vi "Heat_global_variables.vi"() -> ()   [LabVIEW 2019]
uses:
  Monitors/Utility/Monitor Communication/K6221/K6221_Cluster.ctl
panel:
  in  "Bin_file_Heat":refnum<file>
  in  "K6221-Heat-variables":T1
  # "K 6221"
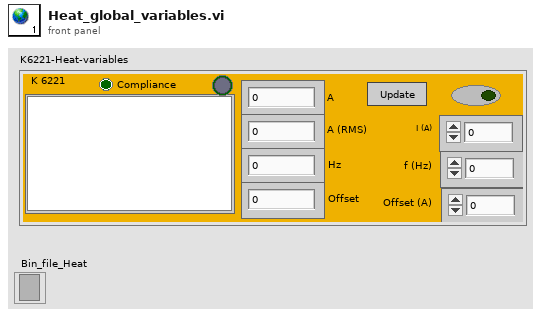
[diagram p1: front panel]
types:
  T1 = typedef "K6221_Cluster.ctl" = cluster{"Plot Window":dbl[][], "A":dbl, "A (RMS)":dbl, "Hz":dbl, "I (A)":dbl, "f (Hz)":dbl, "Update":bool, "Offset":dbl, "Offset (A)":dbl, "Compliance":bool, "Output":bool, "Output Status":bool}
diagram:
